vi "SubVI Rotate Right Gyro.vi"(8 "angle":sgl=85.0, 9 "NXT/EV3":T1, 10 "PortGyro":T2 items=["Port 1", "Port 2", "Port 3", "Port 4"]) -> (2 "NXT/EV3 2":T1)   [LabVIEW 2016]
uses:
  <vilib>/NXT/Subs/LVHSConnector.ctl
  <vilib>/NXT/LegoClasses/BrickReference/BrickReference.lvclass
  <vilib>/NXT/Block Support/NXT_InputPort.ctl
  <vilib>/NXT/Block Support/NXT_OutputPort.ctl
  <vilib>/NXT/Dual Mode Library/Sensors/EV3_Gyro_Angle.vi
  <vilib>/NXT/NXTIO Xnodes/NXTIONodeSubVIs/NXTMoveMotors.vi
  <vilib>/NXT/NXTIO Xnodes/NXTIONodeSubVIs/NXTStopMotors.vi
  <vilib>/NXT/NXTIO Xnodes/AddressXNode/NXTIOAddress.xnode
  <vilib>/NXT/NXTIO Xnodes/NXTIOXNode/NXTIO.xnode
panel:
  in  "angulo0":sgl
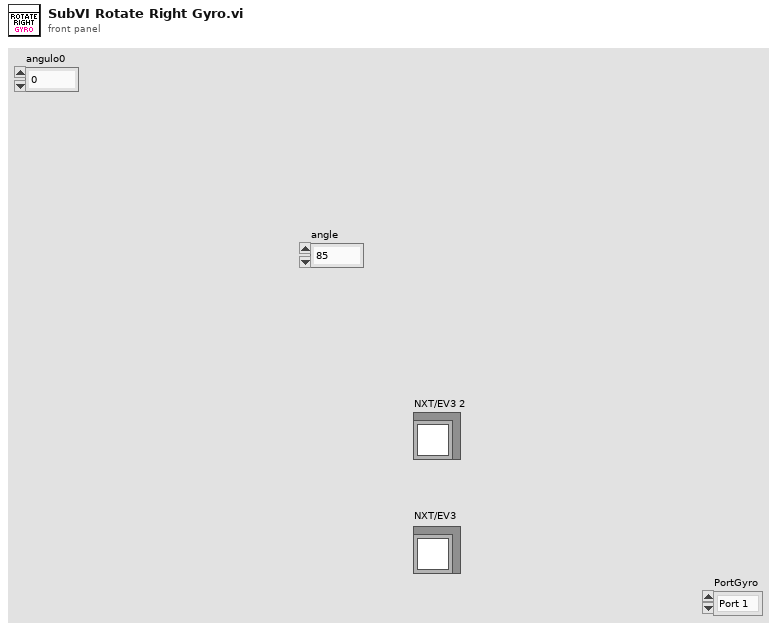
[diagram p1: front panel]
types:
  T1 = typedef "LVHSConnector.ctl" = refnum<class "BrickReference.lvclass">
  T2 = typedef "NXT_InputPort.ctl" = u32
  T3 = typedef "NXT_OutputPort.ctl" = u8
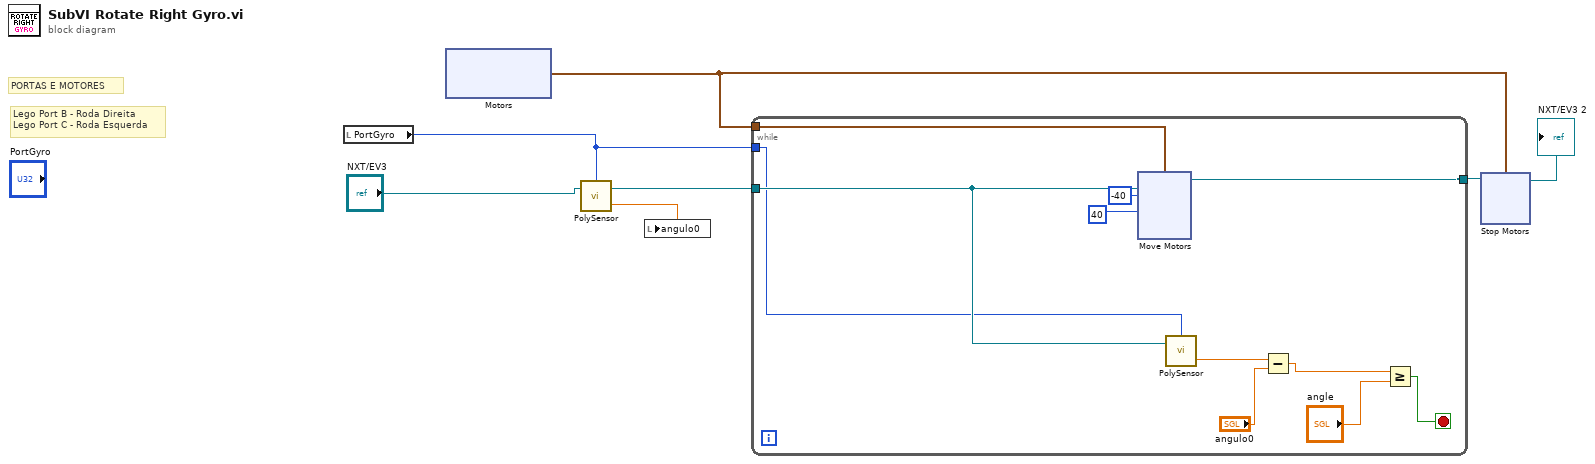
[diagram p0: block diagram]
diagram:
  # "Lego Port B - Roda Direita\nLego Port C - Roda Esquerda"
  # "PORTAS E MOTORES"
  n1 = local read "PortGyro"() -> (w3:T2)
  n2 = xnode "Motors"() -> ("Motor"=w4:cluster{"Port":T3, "Port":T3})
  n3 = call-poly <vilib>:"PolySensor.vi"("NXT/EV3"="NXT/EV3", "Port (Port 1)"=w3) -> ("Degrees"=w6:sgl, "NXT/EV3"=w7:T1)  [unwired: 1 in]
  n4 = local write "angulo0"(w6) -> ()
  n5 = while {
    tunnel: w7 -> [w17]
    tunnel: [w11] -> w5
    tunnel: w4 -> [w10]
    tunnel: w3 -> [w8]
    stop <- w12 stop-if-true
    n6 = xnode "Move Motors"("Power/Speed 1"=i8 -40, "Motors"=w10, "NXT/EV3"=w17, "Power/Speed 2"=i8 40) -> ("NXT/EV3"=w11:T1)
    n7 = call-poly <vilib>:"PolySensor.vi"("NXT/EV3"=w17, "Port (Port 1)"=w8) -> ("Degrees"=w16:sgl)  [unwired: 1 in, 1 out]
    n8 = Subtract(x=w16, y="angulo0") -> (x-y=w14:sgl)
    n9 = Greater Or Equal?(x=w14, y="angle") -> (x >= y?=w12:bool)
  }
  n10 = xnode "Stop Motors"("Motors"=w4, "NXT/EV3"=w5) -> ("NXT/EV3"=→"NXT/EV3 2":T1)
